vi "read project ref.vi"(11 "Builders in":refnum<class "Builder.lvclass">) -> (2 "project ref":refnum<vi>)   [LabVIEW 2024, in "Builder.lvclass"]
uses:
  Builder.lvclass
  Builder.lvclass/Builder.ctl
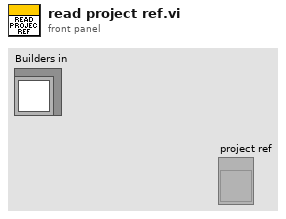
[diagram p1: front panel]
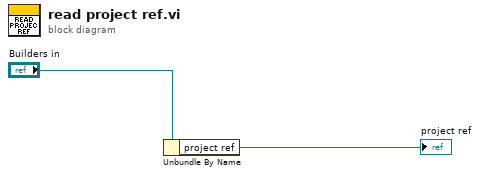
[diagram p0: block diagram]
diagram:
  n1 = Unbundle By Name("Builders in") -> ("project ref"=→"project ref":refnum<vi>)
